vi "Day_File_Plotter.vi"() -> ()   [LabVIEW 2015]
uses:
  Anemometry/Anemometry Sub Vis/File/Setup_Filetype.ctl
panel:
  in  "History (Hours)":i32 min=0
  in  "Use Full Files":bool
  in  "Reload":bool
  out "Setup exists?":bool
  out "Plot 3 status":string
  out "Plot 2 status":string
  out "Plot 1 status":string
  out "Change Scale?":bool
  out "Min Memory":timestamp
  out "Max Memory":timestamp
  in  "Show Full Time?":bool
  in  "Max Time":timestamp format="%<%H:%M\n%x>T"
  in  "Min Time":timestamp format="%<%H:%M\n%x>T"
  out "Plot 3 Chs":string[](array[string])
  out "Plot 2 Chs":string[](array[string])
  out "Plot 1 Chs":string[](array[string])
  in  "Save plot number":T1(ring)
  in  "Data folder location":path
  in  "Save 3":bool
  in  "Save 2":bool
  in  "Save 1":bool
  in  "Averaging Time (min)":dbl=0.01 min=0.0 step=0.01 format="%#.2f"
  in  "End Date":timestamp format="%<%x>T"
  in  "Selector 1":i32[](listbox)
  in  "Search 1":string
  in  "Search 2":string
  in  "Search 3":string
  out "Last Updated":string
  out "Plot 3":cluster{"Times":dbl[], "Output array":dbl[]}[](graph)
  in  "Selector 3":i32[](listbox)
  out "Plot 2":cluster{"Times":dbl[], "Output array":dbl[]}[](graph)
  in  "Selector 2":i32[](listbox)
  in  "stop":bool
  out "Plot 1":cluster{dbl[], "Output array":dbl[]}[](graph)
  in  "History (days)":i32 min=0
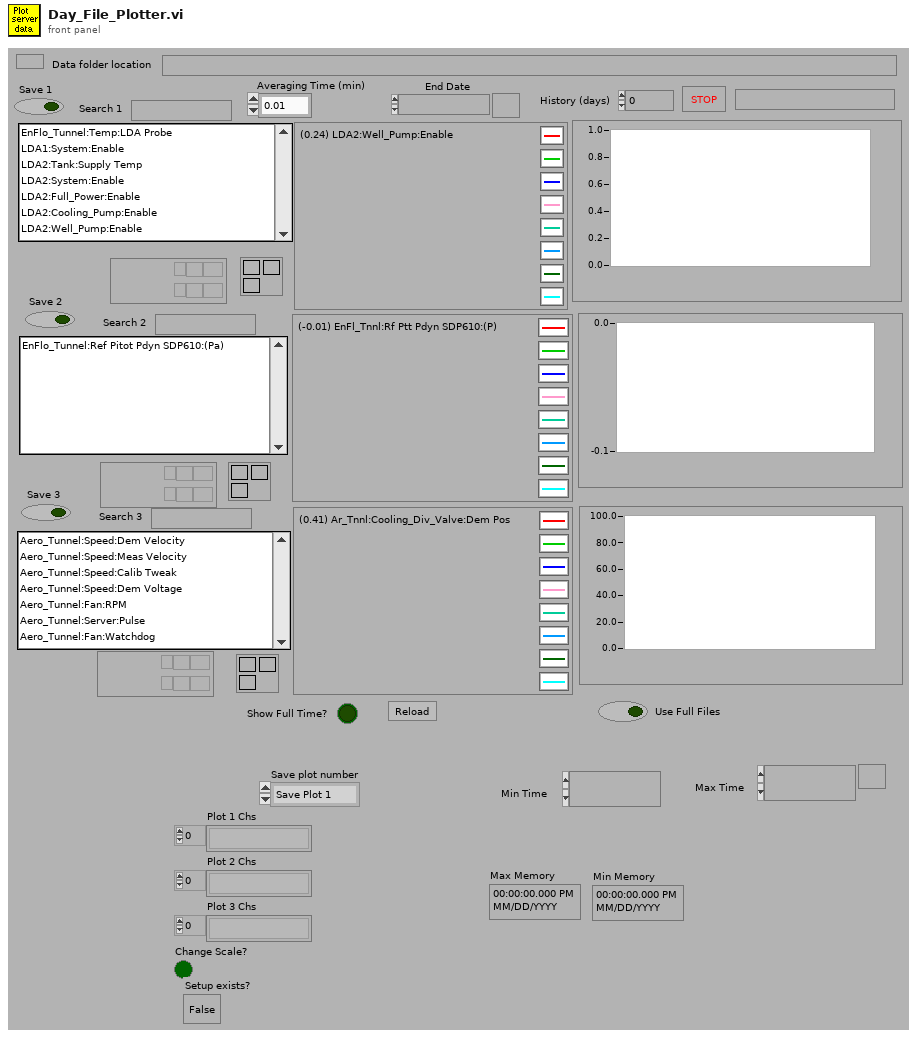
[diagram p1: front panel]
types:
  T1 = enum16{"Save Plot 1", "Save Plot 2", "Save Plot 3"}
  T2 = typedef "Setup_Filetype.ctl" = enum16{"Measurement Setups", "Calibration Setups", "General", "Results File Plotter Setups", "Speed Calib Tweaks"}
  T3 = enum32{"existing file", "new file", "new or existing file", "existing dir", "new dir", "new or existing dir", "existing file (use LLBs)", "new file (use LLBs)", "new or existing file (use LLBs)", "new or existing file or directory (use LLBs)"}
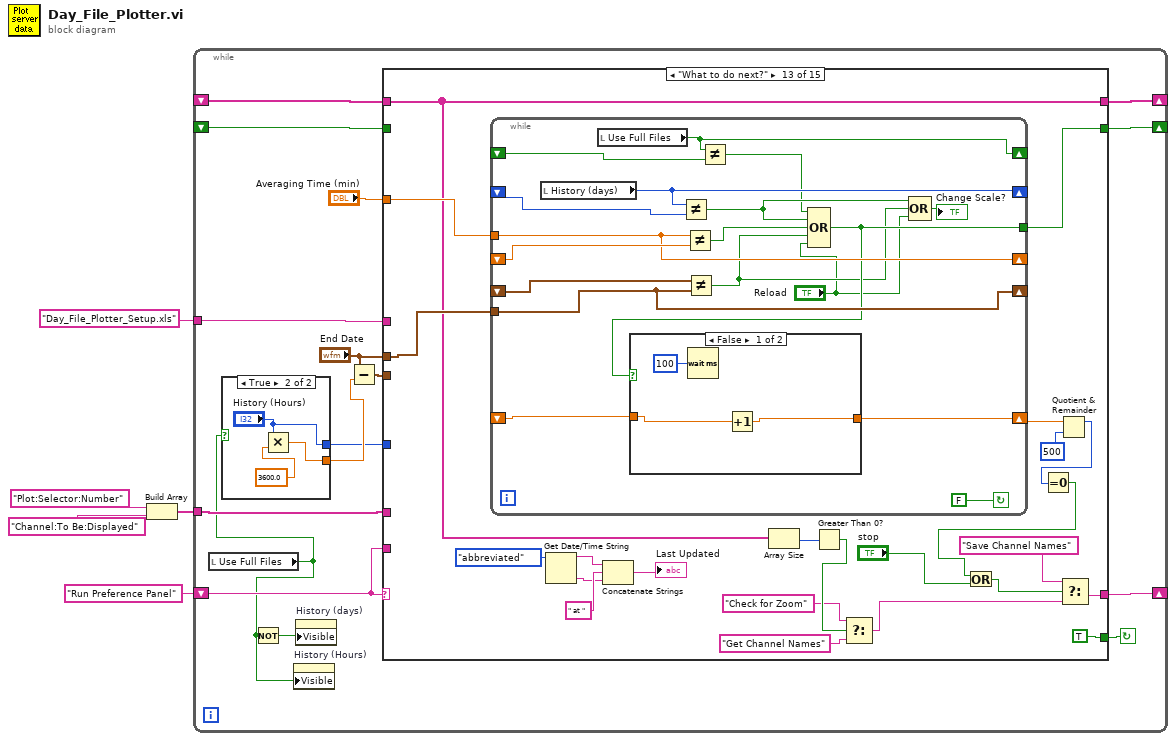
[diagram p0: block diagram]
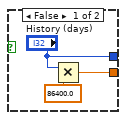
[diagram p2: hidden frame]
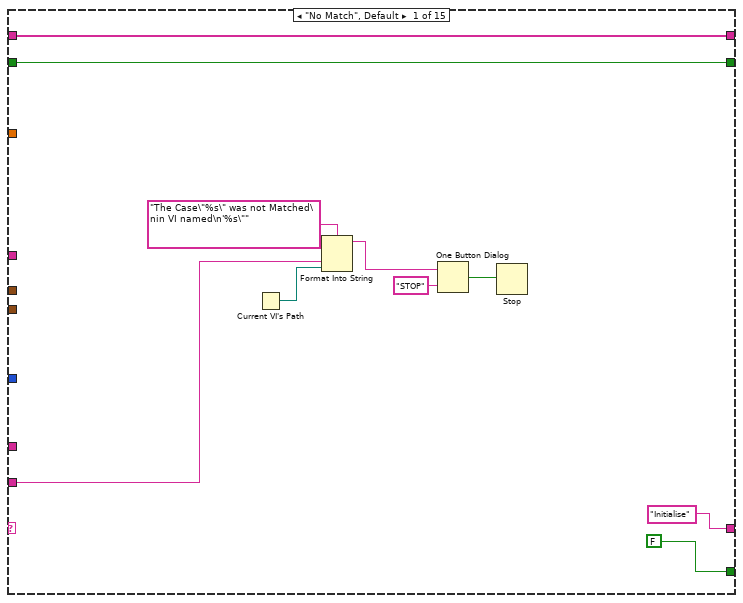
[diagram p3: hidden frame]
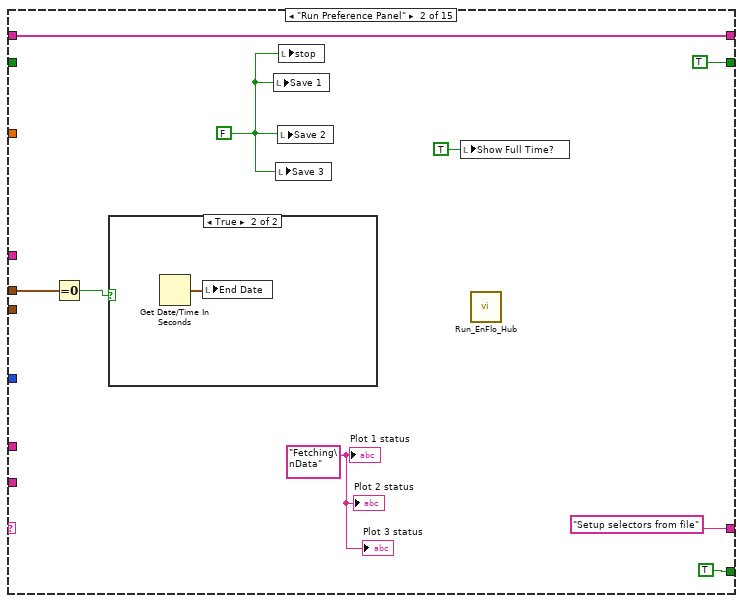
[diagram p4: hidden frame]
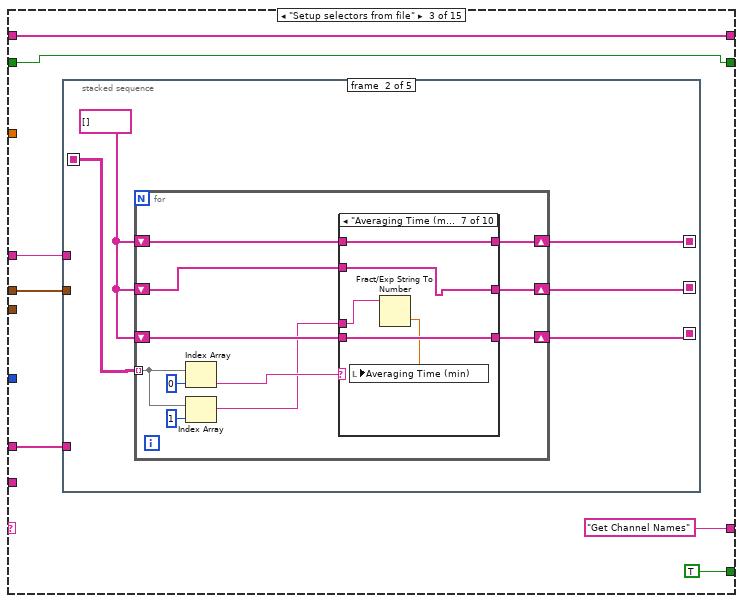
[diagram p6: hidden frame]
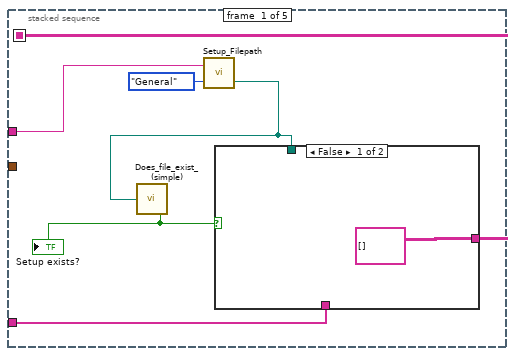
[diagram p7: hidden frame]
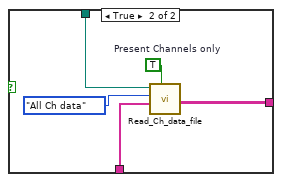
[diagram p8: hidden frame]
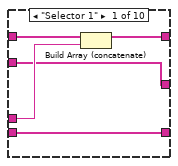
[diagram p9: hidden frame]
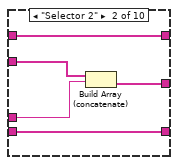
[diagram p10: hidden frame]
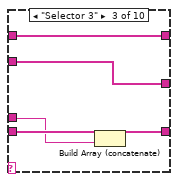
[diagram p11: hidden frame]
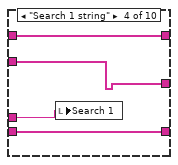
[diagram p12: hidden frame]
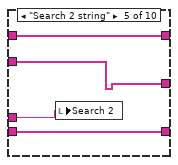
[diagram p13: hidden frame]
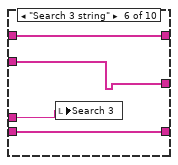
[diagram p14: hidden frame]
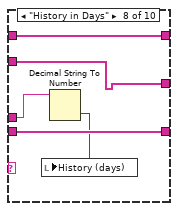
[diagram p15: hidden frame]
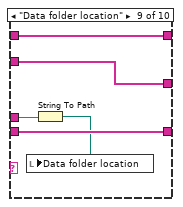
[diagram p16: hidden frame]
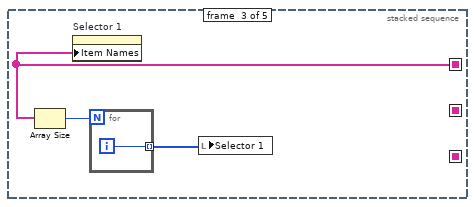
[diagram p18: hidden frame]
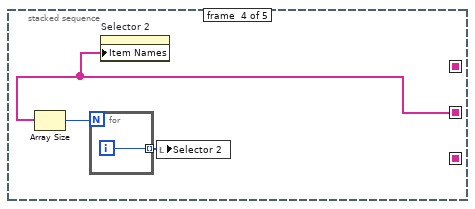
[diagram p19: hidden frame]
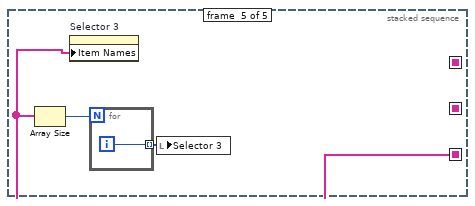
[diagram p20: hidden frame]
diagram:
  n1 = Build Array("Plot:Selector:Number", "Channel:To Be:Displayed") -> (w2:string[])
  n2 = while {
    shift-left: "Run Preference Panel" -> [w19]
    shift-right: [w20] -> _
    tunnel: w2 -> [w18]
    tunnel: "Day_File_Plotter_Setup.xls" -> [w17]
    shift-right: [w13] -> _
    shift-left: _ -> [w12]
    shift-right: [w9] -> _
    shift-left: _ -> [w8]
    stop <- w21 continue-if-true
    n3 = local read "Use Full Files"() -> (w6:bool)
    n4 = case shown="True" w6 {
      tunnel: [w23 w26] -> w16
      tunnel: ["History (days)" "History (Hours)"] -> w11
      frame False {
        n5 = Multiply(x="History (days)", y=86400.0) -> (x*y=w23:dbl)
      }
      frame True {
        n6 = Multiply(x="History (Hours)", y=3600.0) -> (x*y=w26:dbl)
      }
    }
    n7 = Not(x=w6) -> (.not. x?=w7:bool)
    n8 = property on="History (Hours)" class="DigNum (strict)"("Visible"=w6) -> ()  [unwired: 2 in, 2 out]
    n9 = property on="History (days)" class="DigNum (strict)"("Visible"=w7) -> ()  [unwired: 2 in, 2 out]
    n10 = Subtract(x="End Date", y=w16) -> (x-y=w15:timestamp)
    n11 = case shown="\"What to do next?\"" w19 {
      tunnel: [FALSE TRUE TRUE TRUE TRUE TRUE TRUE TRUE TRUE TRUE TRUE TRUE TRUE TRUE w621] -> w21
      tunnel: ["Initialise" "Setup selectors from file" "Get Channel Names" "What to do next?" "Update Plot2?" "Update Plot3?" "Rescale plots?" "Update Plot1?" w325 w377 w431 w483 w579 w605 "Check for Zoom" ("t")] -> w20
      tunnel: w19 -> [w32 _ _ _ _ _ _ _ _ _ _ _ _ _ _]
      tunnel: w18 -> [_ _ w51 _ _ _ _ _ _ _ _ _ _ _ w628]
      tunnel: w17 -> [_ _ w52 _ _ _ _ _ _ _ _ _ _ _ w627]
      tunnel: w15 -> [_ _ _ _ w170 w216 w262 _ _ _ _ _ _ _ _]
      tunnel: "End Date" -> [_ w43 w49 w145 w169 w215 w261 _ _ _ _ _ w572 _ _]
      tunnel: [w29 TRUE w50 w146 w173 w219 w265 w293 w342 w395 w448 w484 w571 w604 w625] -> w13
      tunnel: w12 -> [w29 _ w50 w146 w173 w219 w265 w293 w342 w395 w448 w484 _ w603 w625]
      tunnel: w11 -> [_ _ _ _ _ _ _ _ _ _ _ _ _ _ w619]
      tunnel: "Averaging Time (min)" -> [_ _ _ _ w172 w218 w264 _ _ _ _ _ w570 _ w624]
      tunnel: [w28 w41 w48 w142 w164 w210 w256 w294 w338 w391 w444 w485 w568 w610 w623] -> w9
      tunnel: w8 -> [w28 w41 w48 _ w166 w212 w258 w294 w338 w391 w444 w485 w568 w610 w623]
      frame "No Match", Default {
        n12 = Current VI's Path() -> (path=w31:path)
        n13 = Format Into String(format string="The Case\"%s\" was not Matched\nin VI named\n'%s\"" ("Format String"), w32, w31) -> (resulting string=w35:string)  [unwired: 2 in, 1 out]
        n14 = One Button Dialog(message=w35, button name ("OK")="STOP") -> (true=w33:bool)
        n15 = Stop(stop? (T)=w33) -> ()
      }
      frame "Run Preference Panel" {
        w38 = "Fetching\nData" ("Plot 1 status")
        w40 = FALSE
        n16 = Equal To 0?(x=w43) -> (x = 0?=w42:bool)
        n17 = case shown="True" w42 {
          frame False {
          }
          frame True {
            n18 = Get Date/Time In Seconds() -> (seconds since 1Jan1904=w47:timestamp)
            n19 = local write "End Date"(w47) -> ()
          }
        }
        n20 = local write "Save 1"(w40) -> ()
        n21 = local write "Save 3"(w40) -> ()
        n22 = local write "Save 2"(w40) -> ()
        n23 = local write "stop"(w40) -> ()
        n24 = local write "Show Full Time?"(TRUE ("Show Full Time?")) -> ()
        n25 = call "Run_EnFlo_Hub.vi"() -> ()  [unwired: 8 out]
        "Plot 1 status" <- w38
        "Plot 3 status" <- w38
        "Plot 2 status" <- w38
      }
      frame "Setup selectors from file" {
        n26 = stacked-sequence {
          seq-local: [w59 _ _ _ _] -> [_ w71 _ _ _]
          seq-local: [_ w69 _ _ _] -> [_ _ w130 _ _]
          seq-local: [_ w67 _ _ _] -> [_ _ _ w132 _]
          seq-local: [_ w68 _ _ _] -> [_ _ _ _ w136]
          tunnel: w52 -> [w56 _ _ _ _]
          tunnel: w51 -> [w60 _ _ _ _]
          tunnel: w49 -> [_ _ _ _ _]
          frame #0 {
            n27 = call "Setup_Filepath.vi"("Setup File Type"=Setup_Filetype."General", "Filename in"=w56) -> ("Filename Out"=w55:path)  [unwired: 1 out]
            n28 = call "Does_file_exist_(simple).vi"("Pathname"=w55) -> ("exists?"=w58:bool)
            "Setup exists?" <- w58
            n29 = case shown="False" w58 {
              tunnel: w55 -> [_ w66]
              tunnel: w60 -> [_ w65]
              tunnel: [string[][] [] ("Channel Values") w62] -> w59
              frame False {
              }
              frame True {
                w64 = TRUE  # Present Channels only
                n30 = call "Read_Ch_data_file.vi"("Present Channels only"=w64, "Present Channels"=w65, "Output"=enum16{"All Ch data", "The last few rows"}."All Ch data", "Filename"=w66) -> ("Channel Values"=w62:string[][])  [unwired: 1 in, 4 out]
              }
            }
          }
          frame #1 {
            w70 = string[] []
            n31 = for {
              shift-right: [w77] -> w69
              shift-left: w70 -> [w78]
              tunnel: w71 -> [w79] mode=indexing
              shift-right: [w75] -> w67
              shift-left: w70 -> [w76]
              shift-right: [w73] -> w68
              shift-left: w70 -> [w74]
              n32 = Index Array(array=w79, index=0 ("Index")) -> (element=w81:string)
              n33 = Index Array(array=w79, index=1 ("Index")) -> (element=w72:string)
              n34 = case shown="\"Averaging Time (min)\"" w81 {
                tunnel: w78 -> [w87 w92 w93 w101 w105 w109 w114 w115 w122 w127]
                tunnel: [w86 w92 w93 w101 w105 w109 w114 w115 w122 w127] -> w77
                tunnel: w72 -> [w85 w89 w95 w98 w102 w106 w111 w117 w121 _]
                tunnel: w76 -> [w84 w90 w94 w100 w104 w108 w113 w119 w124 w126]
                tunnel: [w84 w88 w94 w100 w104 w108 w113 w119 w124 w126] -> w75
                tunnel: w74 -> [w83 w91 w97 w99 w103 w107 w112 w118 w123 w125]
                tunnel: [w83 w91 w96 w99 w103 w107 w112 w118 w123 w125] -> w73
                frame "Selector 1" {
                  n35 = Build Array (concatenate)(w87, w85) -> (w86:string[])
                }
                frame "Selector 2" {
                  n36 = Build Array (concatenate)(w90, w89) -> (w88:string[])
                }
                frame "Selector 3" {
                  n37 = Build Array (concatenate)(w97, w95) -> (w96:string[])
                }
                frame "Search 1 string" {
                  n38 = local write "Search 1"(w98) -> ()
                }
                frame "Search 2 string" {
                  n39 = local write "Search 2"(w102) -> ()
                }
                frame "Search 3 string" {
                  n40 = local write "Search 3"(w106) -> ()
                }
                frame "Averaging Time (min)" {
                  n41 = Fract/Exp String To Number(string=w111) -> (number=w110:dbl)  [unwired: 3 in, 1 out]
                  n42 = local write "Averaging Time (min)"(w110) -> ()
                }
                frame "History in Days" {
                  n43 = Decimal String To Number(string=w117) -> (number=w116:i32)  [unwired: 3 out]
                  n44 = local write "History (days)"(w116) -> ()
                }
                frame "Data folder location" {
                  n45 = String To Path(string=w121) -> (path=w120:path)
                  n46 = local write "Data folder location"(w120) -> ()
                }
                frame "No match", Default {
                }
              }
            }
          }
          frame #2 {
            n47 = Array Size(array=w130) -> (size(s)=w129:i32)
            n48 = property on="Selector 1" class="LstBox (strict)"("Item Names"=w130) -> ()  [unwired: 2 in, 2 out]
            n49 = for {
              N: w129 -> [_]
              tunnel: [w131] -> w128 mode=indexing
              i -> [w131]
            }
            n50 = local write "Selector 1"(w128) -> ()
          }
          frame #3 {
            n51 = Array Size(array=w132) -> (size(s)=w134:i32)
            n52 = for {
              N: w134 -> [_]
              tunnel: [w135] -> w133 mode=indexing
              i -> [w135]
            }
            n53 = property on="Selector 2" class="LstBox (strict)"("Item Names"=w132) -> ()  [unwired: 2 in, 2 out]
            n54 = local write "Selector 2"(w133) -> ()
          }
          frame #4 {
            n55 = Array Size(array=w136) -> (size(s)=w138:i32)
            n56 = property on="Selector 3" class="LstBox (strict)"("Item Names"=w136) -> ()  [unwired: 2 in, 2 out]
            n57 = for {
              N: w138 -> [_]
              tunnel: [w139] -> w137 mode=indexing
              i -> [w139]
            }
            n58 = local write "Selector 3"(w137) -> ()
          }
        }
      }
      frame "Get Channel Names" {
        n59 = local read "Setup exists?"() -> (w141:bool)
        n60 = call "Get_Day_File_Client.vi"("Use Full Res Files"="Use Full Files", "End time"=w145, "Start time"=w145, "Channel Names"=string[] ["test"], "Data folder location"="Data folder location") -> ("All Channel Names"=w142:string[])  [unwired: 1 in, 3 out]
        n61 = case shown="False" w141 {
          tunnel: w142 -> [w150 _]
          frame False {
            n62 = local write "Selector 1"(i32[] [0] ("Selector 1")) -> ()
            n63 = property on="Selector 1" class="LstBox (strict)"("Item Names"=w150) -> ()  [unwired: 2 in, 2 out]
          }
          frame True {
          }
        }
      }
      frame "Plot1" {
        n64 = local read "Data folder location"() -> (w171:path)
        n65 = local read "Plot 1 Chs"() -> (w156:string[])
        n66 = local read "Use Full Files"() -> (w151:bool)
        n67 = call "Get_Day_File_Client.vi"("Use Full Res Files"=w151, "Averaging Time (min)"=w172, "End time"=w169, "Start time"=w170, "Channel Names"=w156, "Data folder location"=w171) -> ("All Channel Names"=w165:string[], "Data"=w168:dbl[][], "Times"=w154:dbl[])  [unwired: 1 out]
        n68 = Array Size(array=w165) -> (size(s)=w167:i32)
        n69 = for {
          tunnel: w168 -> [w184] mode=indexing
          tunnel: [w193] -> w163 mode=indexing
          tunnel: w154 -> [w192]
          tunnel: [w188] -> w155 mode=indexing
          tunnel: w156 -> [w185] mode=indexing
          n70 = Bundle("Times"=w192, "Data"=w184) -> (w193:cluster{"Times":dbl[], "Data":dbl[]})  [unwired: 1 out]
          n71 = call "Mean_fr_NaN_data.vi"("Data"=w184) -> ("Mean value"=w183:dbl)  [unwired: 1 out]
          n72 = call "Number_2_string.vi"("precision"="2", "number"=w183) -> ("String"=w186:string)
          n73 = Format Into String(format string="(%s) %s", w186, w185) -> (resulting string=w189:string)  [unwired: 2 in, 1 out]
          n74 = call "Abbreviate_string.vi"("Input String"=w189, "Max String Length"=40) -> ("Output String"=w188:string)
        }
        "Plot 1" <- w163
        n75 = Equal To 0?(x=w167) -> (x = 0?=w153:bool)
        n76 = case shown="False" w153 {
          tunnel: w154 -> [w181 _]
          tunnel: [FALSE ("Visible") FALSE ("Visible")] -> w152
          frame False {
            n77 = Array Max & Min(array=w181) -> (max value=w180:dbl, min value=w178:dbl)  [unwired: 2 out]
            n78 = To Time Stamp(1:w180) -> (0:→"Max Memory":timestamp)
            n79 = To Time Stamp(1:w178) -> (0:→"Min Memory":timestamp)
          }
          frame True {
          }
        }
        n80 = Select(t=w166, s=w153, f=w165) -> (s? t:f=w164:string[])
        n81 = Array Size(array=w155) -> (size(s)=w161:i32)
        n82 = Subtract(x=10 ("dimension size"), y=w161) -> (x-y=w162:i32)
        n83 = Initialize Array("", w162) -> (w159:string[])
        n84 = Build Array (concatenate)(w155, w159) -> (w157:string[])
        n85 = property on="Plot 1 status" class="Str"("Visible"=w152) -> ()  [unwired: 2 in, 2 out]
        n86 = for {
          tunnel: w157 -> [w194] mode=indexing
          i -> [w195]
          n87 = property on="Plot 1" class="XYGraph (strict)"("Active Plot"=w195, "Plot.Plot Name"=w194) -> ()  [unwired: 2 in, 2 out]
        }
      }
      frame "Plot2" {
        n88 = local read "Plot 2 Chs"() -> (w203:string[])
        n89 = local read "Data folder location"() -> (w217:path)
        n90 = local read "Use Full Files"() -> (w196:bool)
        n91 = call "Get_Day_File_Client.vi"("Use Full Res Files"=w196, "Averaging Time (min)"=w218, "End time"=w215, "Start time"=w216, "Channel Names"=w203, "Data folder location"=w217) -> ("All Channel Names"=w211:string[], "Data"=w214:dbl[][], "Times"=w200:dbl[])  [unwired: 1 out]
        n92 = Array Size(array=w211) -> (size(s)=w213:i32)
        n93 = for {
          tunnel: w214 -> [w230] mode=indexing
          tunnel: [w239] -> w202 mode=indexing
          tunnel: w200 -> [w238]
          tunnel: [w234] -> w201 mode=indexing
          tunnel: w203 -> [w231] mode=indexing
          n94 = Bundle("Times"=w238, "Data"=w230) -> (w239:cluster{"Times":dbl[], "Data":dbl[]})  [unwired: 1 out]
          n95 = call "Mean_fr_NaN_data.vi"("Data"=w230) -> ("Mean value"=w229:dbl)  [unwired: 1 out]
          n96 = call "Number_2_string.vi"("precision"="2", "number"=w229) -> ("String"=w232:string)
          n97 = Format Into String(format string="(%s) %s", w232, w231) -> (resulting string=w235:string)  [unwired: 2 in, 1 out]
          n98 = call "Abbreviate_string.vi"("Input String"=w235, "Max String Length"=40) -> ("Output String"=w234:string)
        }
        "Plot 2" <- w202
        n99 = Equal To 0?(x=w213) -> (x = 0?=w199:bool)
        n100 = case shown="True" w199 {
          tunnel: w200 -> [w223 _]
          tunnel: [w222 w228] -> w198
          tunnel: FALSE -> [w222 w228]
          frame False {
            n101 = Array Max & Min(array=w223) -> (max value=w227:dbl, min value=w226:dbl)  [unwired: 2 out]
            n102 = To Time Stamp(1:w227) -> (0:w224:timestamp)
            n103 = To Time Stamp(1:w226) -> (0:w225:timestamp)
            n104 = local write "Max Memory"(w224) -> ()
            n105 = local write "Min Memory"(w225) -> ()
          }
          frame True {
          }
        }
        n106 = Array Size(array=w201) -> (size(s)=w208:i32)
        n107 = Select(t=w212, s=w199, f=w211) -> (s? t:f=w210:string[])
        n108 = Subtract(x=10 ("dimension size"), y=w208) -> (x-y=w209:i32)
        n109 = Initialize Array("", w209) -> (w206:string[])
        n110 = Build Array (concatenate)(w201, w206) -> (w204:string[])
        n111 = property on="Plot 2 status" class="Str"("Visible"=w198) -> ()  [unwired: 2 in, 2 out]
        n112 = for {
          tunnel: w204 -> [w240] mode=indexing
          i -> [w241]
          n113 = property on="Plot 2" class="XYGraph (strict)"("Active Plot"=w241, "Plot.Plot Name"=w240) -> ()  [unwired: 2 in, 2 out]
        }
      }
      frame "Plot3" {
        n114 = local read "Plot 3 Chs"() -> (w249:string[])
        n115 = local read "Data folder location"() -> (w263:path)
        n116 = local read "Use Full Files"() -> (w242:bool)
        n117 = call "Get_Day_File_Client.vi"("Use Full Res Files"=w242, "Averaging Time (min)"=w264, "End time"=w261, "Start time"=w262, "Channel Names"=w249, "Data folder location"=w263) -> ("All Channel Names"=w257:string[], "Data"=w260:dbl[][], "Times"=w246:dbl[])  [unwired: 1 out]
        n118 = Array Size(array=w257) -> (size(s)=w259:i32)
        n119 = for {
          tunnel: w260 -> [w276] mode=indexing
          tunnel: [w285] -> w248 mode=indexing
          tunnel: w246 -> [w284]
          tunnel: [w280] -> w247 mode=indexing
          tunnel: w249 -> [w277] mode=indexing
          n120 = Bundle("Times"=w284, "Data"=w276) -> (w285:cluster{"Times":dbl[], "Data":dbl[]})  [unwired: 1 out]
          n121 = call "Mean_fr_NaN_data.vi"("Data"=w276) -> ("Mean value"=w275:dbl)  [unwired: 1 out]
          n122 = call "Number_2_string.vi"("precision"="2", "number"=w275) -> ("String"=w278:string)
          n123 = Format Into String(format string="(%s) %s", w278, w277) -> (resulting string=w281:string)  [unwired: 2 in, 1 out]
          n124 = call "Abbreviate_string.vi"("Input String"=w281, "Max String Length"=40) -> ("Output String"=w280:string)
        }
        "Plot 3" <- w248
        n125 = Equal To 0?(x=w259) -> (x = 0?=w245:bool)
        n126 = case shown="True" w245 {
          tunnel: w246 -> [w269 _]
          tunnel: [w268 w274] -> w244
          tunnel: FALSE -> [w268 w274]
          frame False {
            n127 = Array Max & Min(array=w269) -> (max value=w273:dbl, min value=w272:dbl)  [unwired: 2 out]
            n128 = To Time Stamp(1:w273) -> (0:w270:timestamp)
            n129 = To Time Stamp(1:w272) -> (0:w271:timestamp)
            n130 = local write "Max Memory"(w270) -> ()
            n131 = local write "Min Memory"(w271) -> ()
          }
          frame True {
          }
        }
        n132 = Array Size(array=w247) -> (size(s)=w254:i32)
        n133 = Select(t=w258, s=w245, f=w257) -> (s? t:f=w256:string[])
        n134 = Subtract(x=10 ("dimension size"), y=w254) -> (x-y=w255:i32)
        n135 = Initialize Array("", w255) -> (w252:string[])
        n136 = Build Array (concatenate)(w247, w252) -> (w250:string[])
        n137 = property on="Plot 3 status" class="Str"("Visible"=w244) -> ()  [unwired: 2 in, 2 out]
        n138 = for {
          tunnel: w250 -> [w286] mode=indexing
          i -> [w287]
          n139 = property on="Plot 3" class="XYGraph (strict)"("Active Plot"=w287, "Plot.Plot Name"=w286) -> ()  [unwired: 2 in, 2 out]
        }
      }
      frame "Check for Zoom" {
        n140 = local read "Change Scale?"() -> (w289:bool)
        n141 = Or(x=w289, y="Show Full Time?") -> (x .or. y?=w288:bool)
        n142 = case shown="False" w288 {
          frame False {
            n143 = local read "Max Time"() -> (w301:timestamp)
            n144 = local read "Min Time"() -> (w302:timestamp)
            n145 = To Double Precision Float(number=w301) -> (double precision float=w300:dbl)
            n146 = To Double Precision Float(number=w302) -> (double precision float=w299:dbl)
            n147 = while {
              tunnel: w300 -> [w311]
              tunnel: w299 -> [w310]
              tunnel: [w304] -> w298
              tunnel: [w303] -> w297
              i -> [w313]
              stop <- w305 continue-if-true
              n148 = Increment(x=w313) -> (x+1=w312:i32)
              n149 = case shown="3" w312 {
                tunnel: [w316 w318 w321] -> w304
                tunnel: [w315 w317 w320] -> w303
                tunnel: [TRUE TRUE FALSE] -> w306
                frame 1, Default {
                  n150 = property on="Plot 1" class="XYGraph (strict)"() -> ("X Scale.Range:Maximum"=w316:dbl, "X Scale.Range:Minimum"=w315:dbl)  [unwired: 2 in, 2 out]
                }
                frame 2 {
                  n151 = property on="Plot 2" class="XYGraph (strict)"() -> ("X Scale.Range:Maximum"=w318:dbl, "X Scale.Range:Minimum"=w317:dbl)  [unwired: 2 in, 2 out]
                }
                frame 3 {
                  n152 = property on="Plot 3" class="XYGraph (strict)"() -> ("X Scale.Range:Maximum"=w321:dbl, "X Scale.Range:Minimum"=w320:dbl)  [unwired: 2 in, 2 out]
                }
              }
              n153 = Equal?(x=w311, y=w304) -> (x = y?=w308:bool)
              n154 = Equal?(x=w303, y=w310) -> (x = y?=w309:bool)
              n155 = And(x=w308, y=w309) -> (x .and. y?=w307:bool)
              n156 = And(x=w307, y=w306) -> (x .and. y?=w305:bool)
            }
            n157 = To Time Stamp(1:w298) -> (0:w295:timestamp)
            n158 = To Time Stamp(1:w297) -> (0:w296:timestamp)
            n159 = local write "Max Time"(w295) -> ()
            n160 = local write "Min Time"(w296) -> ()
          }
          frame True {
          }
        }
      }
      frame "Update Plot1?" {
        n161 = property on="Selector 1" class="LstBox (strict)"() -> ("Item Names"=w336:string[])  [unwired: 2 in, 2 out]
        n162 = case shown="True" "Save 1" {
          tunnel: ["Update Plot2?" "Save Plot" ("t")] -> w323
          frame False {
          }
          frame True {
            n163 = local write "Save plot number"(T1."Save Plot 1" ("Save plot number")) -> ()
          }
        }
        n164 = for {
          tunnel: w338 -> [w365]
          shift-right: [w360] -> w337
          shift-left: string[] [] -> [w361]
          tunnel: w336 -> [w363]
          tunnel: "Selector 1" -> [w362] mode=indexing
          n165 = Index Array(array=w363, index=w362) -> (element=w359:string)
          n166 = Search 1D Array(1D array=w365, element=w359) -> (index of element=w364:i32)  [unwired: 1 out]
          n167 = case shown="0, Default" w364 {
            tunnel: w364 -> [_ _]
            tunnel: w361 -> [w368 w369]
            tunnel: [w367 w369] -> w360
            tunnel: w359 -> [w366 _]
            frame 0, Default {
              n168 = Build Array (concatenate)(w368, w366) -> (w367:string[])
            }
            frame -1 {
            }
          }
        }
        "Plot 1 Chs" <- w337
        n169 = while {
          shift-right: [w370] -> w345
          shift-left: _ -> [w375]
          tunnel: [w375] -> w344
          shift-right: [w372] -> _
          shift-left: _ -> [w373]
          tunnel: w342 -> [w372]
          tunnel: [w371] -> w341
          tunnel: w337 -> [w370]
          stop <- FALSE continue-if-true
          n170 = Not Equal?(x=w373, y=w372) -> (x != y?=w371:bool)
        }
        n171 = Not Equal?(x=w344, y=w345) -> (x != y?=w343:bool)
        n172 = And(x=w342, y=w341) -> (x .and. y?=w340:bool)
        n173 = Compound Arithmetic op=OR(w340, w343) -> (w324:bool)
        n174 = case shown="True" w324 {
          tunnel: [w347 "Plot1"] -> w325
          tunnel: w323 -> [w347 _]
          frame False {
          }
          frame True {
            n175 = property on="Plot 1 status" class="Str"("Visible"=TRUE) -> ()  [unwired: 2 in, 2 out]
          }
        }
        n176 = call "Selection_with_Search.vi"("Selected Channel Names"=w337, "Search String"="Search 1", "All Channel Names"=w338) -> ("Item Names"=w333:string[])
        n177 = for {
          tunnel: w333 -> [w358]
          tunnel: w337 -> [w357] mode=indexing
          tunnel: [w356] -> w334 mode=indexing
          n178 = Search 1D Array(1D array=w358, element=w357) -> (index of element=w356:i32)  [unwired: 1 out]
        }
        n179 = Not Equal?(x=w333, y=w336) -> (x != y?=w335:bool)
        n180 = To Double Precision Float(number="Max Time") -> (double precision float=w328:dbl)
        n181 = To Double Precision Float(number="Min Time") -> (double precision float=w326:dbl)
        n182 = case shown="True" w335 {
          tunnel: w334 -> [_ w355]
          tunnel: w333 -> [_ w354]
          frame False {
          }
          frame True {
            n183 = local write "Selector 1"(w355) -> ()
            n184 = property on="Selector 1" class="LstBox (strict)"("Item Names"=w354, "Top Row"=0) -> ()  [unwired: 2 in, 2 out]
          }
        }
        n185 = property on="Plot 1" class="XYGraph (strict)"("X Scale.Range:Maximum"=w328, "X Scale.Range:Minimum"=w326) -> ()  [unwired: 2 in, 2 out]
      }
      frame "Update Plot2?" {
        n186 = property on="Selector 2" class="LstBox (strict)"() -> ("Item Names"=w386:string[])  [unwired: 2 in, 2 out]
        n187 = case shown="True" "Save 2" {
          tunnel: ["Update Plot3?" "Save Plot" ("t")] -> w376
          frame False {
          }
          frame True {
            n188 = local write "Save plot number"(T1."Save Plot 2" ("Save plot number")) -> ()
          }
        }
        n189 = for {
          tunnel: w391 -> [w418]
          shift-right: [w413] -> w390
          shift-left: string[] [] -> [w414]
          tunnel: w386 -> [w416]
          tunnel: "Selector 2" -> [w415] mode=indexing
          n190 = Index Array(array=w416, index=w415) -> (element=w412:string)
          n191 = Search 1D Array(1D array=w418, element=w412) -> (index of element=w417:i32)  [unwired: 1 out]
          n192 = case shown="0, Default" w417 {
            tunnel: w417 -> [_ _]
            tunnel: w414 -> [w421 w422]
            tunnel: [w420 w422] -> w413
            tunnel: w412 -> [w419 _]
            frame 0, Default {
              n193 = Build Array (concatenate)(w421, w419) -> (w420:string[])
            }
            frame -1 {
            }
          }
        }
        "Plot 2 Chs" <- w390
        n194 = while {
          shift-right: [w423] -> w398
          shift-left: _ -> [w428]
          tunnel: [w428] -> w397
          shift-right: [w425] -> _
          shift-left: _ -> [w426]
          tunnel: w395 -> [w425]
          tunnel: [w424] -> w394
          tunnel: w390 -> [w423]
          stop <- FALSE continue-if-true
          n195 = Not Equal?(x=w426, y=w425) -> (x != y?=w424:bool)
        }
        n196 = Not Equal?(x=w397, y=w398) -> (x != y?=w396:bool)
        n197 = And(x=w395, y=w394) -> (x .and. y?=w393:bool)
        n198 = local read "Max Time"() -> (w381:timestamp)
        n199 = local read "Min Time"() -> (w382:timestamp)
        n200 = Compound Arithmetic op=OR(w393, w396) -> (w378:bool)
        n201 = To Double Precision Float(number=w381) -> (double precision float=w380:dbl)
        n202 = To Double Precision Float(number=w382) -> (double precision float=w379:dbl)
        n203 = case shown="True" w378 {
          tunnel: [w400 "Plot2"] -> w377
          tunnel: w376 -> [w400 _]
          frame False {
          }
          frame True {
            n204 = property on="Plot 2 status" class="Str"("Visible"=TRUE) -> ()  [unwired: 2 in, 2 out]
          }
        }
        n205 = call "Selection_with_Search.vi"("Selected Channel Names"=w390, "Search String"="Search 2", "All Channel Names"=w391) -> ("Item Names"=w387:string[])
        n206 = for {
          tunnel: w387 -> [w411]
          tunnel: w390 -> [w410] mode=indexing
          tunnel: [w409] -> w388 mode=indexing
          n207 = Search 1D Array(1D array=w411, element=w410) -> (index of element=w409:i32)  [unwired: 1 out]
        }
        n208 = property on="Plot 2" class="XYGraph (strict)"("X Scale.Range:Maximum"=w380, "X Scale.Range:Minimum"=w379) -> ()  [unwired: 2 in, 2 out]
        n209 = Not Equal?(x=w387, y=w386) -> (x != y?=w389:bool)
        n210 = case shown="True" w389 {
          tunnel: w388 -> [_ w408]
          tunnel: w387 -> [_ w407]
          frame False {
          }
          frame True {
            n211 = property on="Selector 2" class="LstBox (strict)"("Item Names"=w407, "Top Row"=0) -> ()  [unwired: 2 in, 2 out]
            n212 = local write "Selector 2"(w408) -> ()
          }
        }
      }
      frame "Update Plot3?" {
        n213 = property on="Selector 3" class="LstBox (strict)"() -> ("Item Names"=w436:string[])  [unwired: 2 in, 2 out]
        n214 = case shown="False" "Save 3" {
          tunnel: ["Rescale plots?" "Save Plot" ("t")] -> w429
          frame False {
          }
          frame True {
            n215 = local write "Save plot number"(T1."Save Plot 3" ("Save plot number")) -> ()
          }
        }
        n216 = for {
          tunnel: w444 -> [w471]
          shift-right: [w466] -> w443
          shift-left: string[] [] -> [w467]
          tunnel: w436 -> [w469]
          tunnel: "Selector 3" -> [w468] mode=indexing
          n217 = Index Array(array=w469, index=w468) -> (element=w465:string)
          n218 = Search 1D Array(1D array=w471, element=w465) -> (index of element=w470:i32)  [unwired: 1 out]
          n219 = case shown="0, Default" w470 {
            tunnel: w470 -> [_ _]
            tunnel: w467 -> [w474 w475]
            tunnel: [w473 w475] -> w466
            tunnel: w465 -> [w472 _]
            frame 0, Default {
              n220 = Build Array (concatenate)(w474, w472) -> (w473:string[])
            }
            frame -1 {
            }
          }
        }
        "Plot 3 Chs" <- w443
        n221 = while {
          shift-right: [w476] -> w451
          shift-left: _ -> [w481]
          tunnel: [w481] -> w450
          shift-right: [w478] -> _
          shift-left: _ -> [w479]
          tunnel: w448 -> [w478]
          tunnel: [w477] -> w447
          tunnel: w443 -> [w476]
          stop <- FALSE continue-if-true
          n222 = Not Equal?(x=w479, y=w478) -> (x != y?=w477:bool)
        }
        n223 = Not Equal?(x=w450, y=w451) -> (x != y?=w449:bool)
        n224 = And(x=w448, y=w447) -> (x .and. y?=w446:bool)
        n225 = Compound Arithmetic op=OR(w446, w449) -> (w430:bool)
        n226 = case shown="True" w430 {
          tunnel: [w453 "Plot3"] -> w431
          tunnel: w429 -> [w453 _]
          frame False {
          }
          frame True {
            n227 = property on="Plot 3 status" class="Str"("Visible"=TRUE) -> ()  [unwired: 2 in, 2 out]
          }
        }
        n228 = local read "Max Time"() -> (w434:timestamp)
        n229 = local read "Min Time"() -> (w435:timestamp)
        n230 = call "Selection_with_Search.vi"("Selected Channel Names"=w443, "Search String"="Search 3", "All Channel Names"=w444) -> ("Item Names"=w440:string[])
        n231 = for {
          tunnel: w440 -> [w464]
          tunnel: w443 -> [w463] mode=indexing
          tunnel: [w462] -> w441 mode=indexing
          n232 = Search 1D Array(1D array=w464, element=w463) -> (index of element=w462:i32)  [unwired: 1 out]
        }
        n233 = Not Equal?(x=w440, y=w436) -> (x != y?=w442:bool)
        n234 = To Double Precision Float(number=w434) -> (double precision float=w433:dbl)
        n235 = To Double Precision Float(number=w435) -> (double precision float=w432:dbl)
        n236 = case shown="True" w442 {
          tunnel: w441 -> [_ w461]
          tunnel: w440 -> [_ w460]
          frame False {
          }
          frame True {
            n237 = local write "Selector 3"(w461) -> ()
            n238 = property on="Selector 3" class="LstBox (strict)"("Item Names"=w460, "Top Row"=0) -> ()  [unwired: 2 in, 2 out]
          }
        }
        n239 = property on="Plot 3" class="XYGraph (strict)"("X Scale.Range:Maximum"=w433, "X Scale.Range:Minimum"=w432) -> ()  [unwired: 2 in, 2 out]
      }
      frame "Save Plot" {
        n240 = stacked-sequence {
          seq-local: [w500 _] -> [_ w536]
          seq-local: [w488 _] -> [_ w538]
          seq-local: [w486 _] -> [_ w537]
          tunnel: ["What to do next?" _] -> w483
          frame #0 {
            n241 = case shown="\"Save Plot 3\"" "Save plot number" {
              tunnel: [w513 w516 w519] -> w505
              tunnel: [w512 w515 w518] -> w500
              frame "Save Plot 1" {
                n242 = local read "Plot 1 Chs"() -> (w512:string[])
                n243 = local write "Save 1"(FALSE ("Save 1")) -> ()
                n244 = local read "Plot 1"() -> (w513:cluster{dbl[], "Output array":dbl[]}[])
              }
              frame "Save Plot 2" {
                n245 = local read "Plot 2 Chs"() -> (w515:string[])
                n246 = local write "Save 2"(FALSE ("Save 1")) -> ()
                n247 = local read "Plot 2"() -> (w516:cluster{"Times":dbl[], "Output array":dbl[]}[])
              }
              frame "Save Plot 3" {
                n248 = local read "Plot 3 Chs"() -> (w518:string[])
                n249 = local write "Save 3"(FALSE ("Save 1")) -> ()
                n250 = local read "Plot 3"() -> (w519:cluster{"Times":dbl[], "Output array":dbl[]}[])
              }
            }
            n251 = local read "Min Time"() -> (w499:timestamp)
            n252 = local read "Max Time"() -> (w497:timestamp)
            n253 = Index Array(array=w505, index=0) -> (element=w503:cluster{"Times":dbl[], "Output array":dbl[]})
            n254 = To Double Precision Float(number=w499) -> (double precision float=w495:dbl)
            n255 = To Double Precision Float(number=w497) -> (double precision float=w496:dbl)
            n256 = Unbundle(w503) -> ("Times"=w489:dbl[])  [unwired: 1 out]
            n257 = Threshold 1D Array(2:w495, 3:w489) -> (0:w498:dbl)  [unwired: 1 out]
            n258 = Threshold 1D Array(2:w496, 3:w489) -> (0:w494:dbl)  [unwired: 1 out]
            n259 = Round Toward -Infinity(1:w498) -> (0:w492:dbl)
            n260 = Round Toward +Infinity(x=w494) -> (ceil(x): smallest int >= x=w493:dbl)
            n261 = To Long Integer(number=w492) -> (32bit integer=w491:i32)
            n262 = Subtract(x=w493, y=w492) -> (x-y=w490:dbl)
            n263 = for {
              N: w490 -> [_]
              tunnel: w491 -> [w510]
              tunnel: w489 -> [w508]
              tunnel: [w507] -> w488 mode=indexing
              tunnel: [w506] -> w487 mode=indexing
              i -> [w509]
              n264 = Add(x=w510, y=w509) -> (x+y=w506:i32)
              n265 = Index Array(array=w508, index=w506) -> (element=w507:dbl)
            }
            n266 = for {
              tunnel: w505 -> [w523] mode=indexing
              tunnel: w487 -> [w522]
              tunnel: [w520] -> w486 mode=indexing
              n267 = Unbundle(w523) -> ("Output array"=w521:dbl[])  [unwired: 1 out]
              n268 = for {
                tunnel: w522 -> [w526] mode=indexing
                tunnel: w521 -> [w525]
                tunnel: [w524] -> w520 mode=indexing
                n269 = Index Array(array=w525, index=w526) -> (element=w524:dbl)
              }
            }
          }
          frame #1 {
            w531 = FALSE  # append to file? (new file:F)
            (unwired) T3."new file" ("select mode (2)")
            n270 = for {
              tunnel: w537 -> [w555]
              tunnel: w538 -> [w549] mode=indexing
              tunnel: [w551] -> w530 mode=indexing
              i -> [w554]
              n271 = Number To Decimal String(number=w549) -> (decimal integer string=w550:string)  [unwired: 1 out]
              n272 = Index Array(array=w555, index (col)=w554) -> (element=w553:dbl[])  [unwired: 1 in]
              n273 = Get Date/Time String(seconds (now)=w549) -> (date string=w548:string, time string=w547:string)  [unwired: 2 out]
              n274 = for {
                tunnel: w553 -> [w557] mode=indexing
                tunnel: [w556] -> w552 mode=indexing
                n275 = call "Number_2_string.vi"("number"=w557) -> ("String"=w556:string)  [unwired: 1 in]
              }
              n276 = Build Array (concatenate)(w548, w547, w550, w552) -> (w551:string[])
            }
            n277 = Build Array (concatenate)("Date::", "Centre:Time:", "Seconds:Since:1st Jan 1904", w536) -> (w529:string[])
            n278 = call "Ch_names_to_rows.vi"("Channel Names"=w529) -> ("3 Row names"=w535:string[][])
            n279 = File Dialog(7:"Please choose file name" ("prompt")) -> (3:w543:path)  [unwired: 1 in, 8 out]
            n280 = Build Array (concatenate)(w535, w530) -> (w533:string[][])
            n281 = Strip Path(path=w543) -> (stripped path=w540:path, name=w542:string)
            n282 = call "Add_filename_suffix.vi"("Filename"=w542, "Suffix to add"=".xls") -> ("Filename out"=w539:string)  [unwired: 3 out]
            n283 = Array To Spreadsheet String(array=w533, 3:"%s" ("format string")) -> (spreadsheet string=w532:string)  [unwired: 1 out]
            n284 = Build Path(base path=w540, name or relative path=w539) -> (appended path=w528:path)
            n285 = call "Write_File_Simple.vi"("append to file? (new file:F)"=w531, "character string"=w532, "file path"=w528) -> ()  [unwired: 2 out]
          }
        }
      }
      frame "What to do next?" {
        n286 = while {
          shift-right: [w598] -> _
          shift-left: _ -> [w597]
          shift-right: [w594] -> _
          shift-left: _ -> [w595]
          tunnel: w570 -> [w594]
          shift-right: [w592] -> _
          shift-left: _ -> [w593]
          tunnel: w572 -> [w592]
          tunnel: [w590] -> w571
          shift-right: [w588] -> w562
          shift-left: _ -> [w589]
          shift-right: [w582] -> _
          shift-left: _ -> [w583]
          stop <- FALSE continue-if-true
          n287 = local read "History (days)"() -> (w598:i32)
          n288 = local read "Use Full Files"() -> (w582:bool)
          n289 = Not Equal?(x=w598, y=w597) -> (x != y?=w587:bool)
          n290 = Not Equal?(x=w594, y=w595) -> (x != y?=w591:bool)
          n291 = Not Equal?(x=w593, y=w592) -> (x != y?=w586:bool)
          n292 = Not Equal?(x=w582, y=w583) -> (x != y?=w581:bool)
          n293 = Compound Arithmetic op=OR(w581, w587, w591, w586, "Reload") -> (w590:bool)
          n294 = case shown="False" w590 {
            tunnel: w589 -> [w599 w602]
            tunnel: [w600 w602] -> w588
            frame False {
              n295 = Wait (ms)(milliseconds to wait=u32 100) -> ()  [unwired: 1 out]
              n296 = Increment(x=w599) -> (x+1=w600:dbl)
            }
            frame True {
            }
          }
          n297 = Compound Arithmetic op=OR(w587, w586, "Reload") -> (→"Change Scale?":bool)
        }
        n298 = Get Date/Time String(date format (0)=enum16{"short", "long", "abbreviated"}."abbreviated") -> (date string=w575:string, time string=w576:string)  [unwired: 2 out]
        n299 = Concatenate Strings(w575, " at " ("Substring"), w576) -> (→"Last Updated":string)
        n300 = Array Size(array=w568) -> (size(s)=w569:i32)
        n301 = Greater Than 0?(x=w569) -> (x > 0?=w567:bool)
        n302 = Select(t="Check for Zoom", s=w567, f="Get Channel Names") -> (s? t:f=w564:string)
        n303 = Quotient & Remainder(x=w562, y=500) -> (x-y*floor(x/y)=w561:i32)  [unwired: 1 out]
        n304 = Equal To 0?(x=w561) -> (x = 0?=w559:bool)
        n305 = Or(x=w559, y="stop") -> (x .or. y?=w558:bool)
        n306 = Select(t="Save Channel Names", s=w558, f=w564) -> (s? t:f=w579:string)
      }
      frame "Rescale plots?" {
        n307 = local read "Show Full Time?"() -> (w606:bool)
        n308 = local read "Change Scale?"() -> (w608:bool)
        n309 = Or(x=w608, y=w606) -> (x .or. y?=w607:bool)
        n310 = case shown="False" w607 {
          tunnel: ["What to do next?" "Update Plot1?"] -> w605
          tunnel: [w611 FALSE] -> w604
          tunnel: w603 -> [w611 _]
          frame False {
          }
          frame True {
            w614 = FALSE ("Show Full Time?")
            n311 = local write "Show Full Time?"(w614) -> ()
            n312 = local write "Change Scale?"(w614) -> ()
            n313 = local read "Max Memory"() -> (w616:timestamp)
            n314 = local read "Min Memory"() -> (w617:timestamp)
            n315 = local write "Max Time"(w616) -> ()
            n316 = local write "Min Time"(w617) -> ()
          }
        }
      }
      frame "Save Channel Names" {
        w618 = 10 ("y")
        n317 = Less?(x=w619, y=w618) -> (x < y?=w620:bool)
        n318 = stacked-sequence {
          seq-local: [w630 _ _] -> [_ w673 _]
          seq-local: [_ w670 _] -> [_ _ w684]
          tunnel: w628 -> [_ _ w685]
          tunnel: w627 -> [_ _ w681]
          tunnel: w624 -> [_ w669 _]
          tunnel: w620 -> [_ w657 _]
          tunnel: w619 -> [_ w656 _]
          tunnel: w618 -> [_ w655 _]
          frame #0 {
            n319 = for {
              N: 3 -> [_]
              shift-right: [w634] -> w630
              shift-left: string[][] [] -> [w636]
              i -> [w641]
              n320 = Increment(x=w641) -> (x+1=w638:i32)
              n321 = case shown="2" w638 {
                tunnel: [w648 w649 w651] -> w640
                tunnel: [w647 w650 w652] -> w632
                frame 1, Default {
                  n322 = local read "Selector 1"() -> (w648:i32[])
                  n323 = property on="Selector 1" class="LstBox (strict)"() -> ("Item Names"=w647:string[])  [unwired: 2 in, 2 out]
                }
                frame 2 {
                  n324 = property on="Selector 2" class="LstBox (strict)"() -> ("Item Names"=w650:string[])  [unwired: 2 in, 2 out]
                  n325 = local read "Selector 2"() -> (w649:i32[])
                }
                frame 3 {
                  n326 = local read "Selector 3"() -> (w651:i32[])
                  n327 = property on="Selector 3" class="LstBox (strict)"() -> ("Item Names"=w652:string[])  [unwired: 2 in, 2 out]
                }
              }
              n328 = Format Into String(format string="%d" ("Format String"), initial string="Selector ", w638) -> (resulting string=w635:string)  [unwired: 1 in, 1 out]
              n329 = for {
                tunnel: w640 -> [w646] mode=indexing
                tunnel: w635 -> [w645]
                tunnel: [w643] -> w633 mode=indexing
                tunnel: w632 -> [w642]
                n330 = Index Array(array=w642, index=w646) -> (element=w644:string)
                n331 = Build Array(w645, w644) -> (w643:string[])
              }
              n332 = Build Array (concatenate)(w636, w633) -> (w634:string[][])
            }
          }
          frame #1 {
            n333 = Select(t=w656, s=w657, f=w655) -> (s? t:f=w654:i32)
            n334 = local read "Data folder location"() -> (w660:path)
            n335 = local read "Search 1"() -> (w679:string)
            n336 = Number To Fractional String(number=w669, precision (6)=i16 2) -> (F-format string=w667:string)  [unwired: 2 in]
            n337 = local read "Search 2"() -> (w676:string)
            n338 = Number To Decimal String(number=w654) -> (decimal integer string=w664:string)  [unwired: 1 out]
            n339 = local read "Search 3"() -> (w675:string)
            n340 = Path To String(path=w660) -> (string=w659:string)
            n341 = Build Array("Averaging Time (min)" ("element"), w667) -> (w665:string[])
            n342 = Build Array("Search 1 string" ("element"), w679) -> (w666:string[])
            n343 = Build Array("History in Days" ("element"), w664) -> (w662:string[])
            n344 = Build Array("Search 2 string" ("element"), w676) -> (w672:string[])
            n345 = Build Array("Search 3 string" ("element"), w675) -> (w671:string[])
            n346 = Build Array("Data folder location", w659) -> (w658:string[])
            n347 = Build Array (concatenate)(w673, w658, w662, w665, w666, w672, w671) -> (w670:string[][])
          }
          frame #2 {
            n348 = call "Setup_Filepath.vi"("Setup File Type"=Setup_Filetype."General", "Filename in"=w681) -> ("Filename Out"=w680:path)  [unwired: 1 out]
            n349 = Array Size(array=w684) -> (size(s)=w687:i32[])
            n350 = Index Array(array=w687, index=1 ("Index")) -> (element=w686:i32)
            n351 = Not Equal To 0?(x=w686) -> (x != 0?=w683:bool)
            n352 = case shown="True" w683 {
              tunnel: w680 -> [w689 w694]
              tunnel: w684 -> [_ w695]
              tunnel: w685 -> [_ w696]
              frame False {
                n353 = Delete(path (use dialog)=w689) -> ()  [unwired: 1 in, 6 out]
              }
              frame True {
                w690 = FALSE  # append to file? (new file:F)
                n354 = call "Ch_names_to_rows.vi"("Channel Names"=w696) -> ("3 Row names"=w697:string[][])
                n355 = Build Array (concatenate)(w697, w695) -> (w692:string[][])
                n356 = Array To Spreadsheet String(array=w692, 3:"%s" ("format string")) -> (spreadsheet string=w691:string)  [unwired: 1 out]
                n357 = call "Write_File_Simple.vi"("append to file? (new file:F)"=w690, "character string"=w691, "file path"=w694) -> ()  [unwired: 2 out]
              }
            }
          }
        }
        n358 = local read "stop"() -> (w622:bool)
        n359 = Not(x=w622) -> (.not. x?=w621:bool)
      }
    }
  }
